vi "TX OOB Test Cases.vi"() -> (0 "error out":errorcluster, 2 "status":string, 3 "pass":bool)   [LabVIEW 2021]
uses:
  Common/Typedef/Plugin Status.ctl
  Common/Typedef/Plugin State.ctl
  Common/Typedef/Timing Statistics.ctl
  Common/Typedef/Timing Stats Base.ctl
  Common/Typedef/FIFO Statistics.ctl
  Common/Typedef/Simple Error.ctl
  Common/Typedef/Monitor Doubles.ctl
  Common/Typedef/Monitor U64.ctl
  Common/Typedef/Monitor I64.ctl
  CIFUtilities/CIFOutOfBand/CIFOutOfBand.lvclass/CIFOutOfBand.ctl
  OOB_Tx/Typedef/OOB Core Commands.ctl
  Common/Typedef/Plugin Overrides.ctl
  Common/Typedef/Timing Overrides.ctl
  CIFUtilities/CIFChannelMng/typedef/Channel List for OOB.ctl
  CIFUtilities/CIFChannels/Typedef/Direction.ctl
  OOB_Tx/Private/Command Settings.vi
  CIFUtilities/CIFOutOfBand/Accessors/Write Local OOB Data.vi
  CIFUtilities/CIFOutOfBand/Write OOB DVR.vi
  CIFUtilities/CIFOutOfBand/Utilities/Command to Bitwise Command.vi
  CIFUtilities/CIFOutOfBand/Accessors/Read Local OOB Data.vi
  CIFUtilities/CIFOutOfBand/Read OOB DVR.vi
  OOB_Tx/Private/Read Payload.vi
  OOB_Tx/CIFCoreOOB_Tx.lvclass
  D:/dev/CIF-LVCore/src/CIFUtilities/CIFOutOfBand/CIFOutOfBand.lvclass
  CIFUtilities/CIFOutOfBand/Init OOB.vi
  CIFUtilities/CIFOutOfBand/CIFOutOfBand.lvclass
  Common/CIFCoreCommon.lvlib
  CIFUtilities/CIFChannels/CIFChannels.lvclass
  CIFUtilities/CIFChannelMng/CIFChannelMng.lvclass
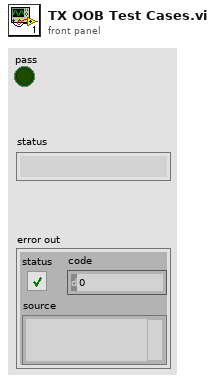
[diagram p1: front panel]
types:
  T1 = typedef "CIFCoreCommon.lvlib/Plugin Status.ctl" = cluster{"State":T2, "Timing Statistics (us)":T3, "FIFO Statistics (us)":T5, "error":T6, "Monitor Doubles":T7, "Monitor U64":T8, "Monitor I64":T9, "Cleanup":T4, "Create":i32, "Destroy":i32}
  T2 = typedef "CIFCoreCommon.lvlib/Plugin State.ctl" = enum32{"Null", "Creating", "Listening", "Running", "CleaningUp", "Destroying"}
  T3 = typedef "CIFCoreCommon.lvlib/Timing Statistics.ctl" = cluster{"Period":T4, "Wake Error":T4, "Execute":T4, "Housekeep":T4, "Idle":T4}
  T4 = typedef "CIFCoreCommon.lvlib/Timing Stats Base.ctl" = cluster{"Max":i32, "Min":i32}
  T5 = typedef "CIFCoreCommon.lvlib/FIFO Statistics.ctl" = cluster{"From T0":T4, "From Previous Plugin":T4, "Output Error":T4}
  T6 = typedef "CIFCoreCommon.lvlib/Simple Error.ctl" = cluster{"status":bool, "code":i32}
  T7 = typedef "CIFCoreCommon.lvlib/Monitor Doubles.ctl" = cluster{"1":dbl, "2":dbl, "3":dbl, "4":dbl}
  T8 = typedef "CIFCoreCommon.lvlib/Monitor U64.ctl" = cluster{"1":u64, "2":u64, "3":u64, "4":u64}
  T9 = typedef "CIFCoreCommon.lvlib/Monitor I64.ctl" = cluster{"1":i64, "2":i64, "3":i64, "4":i64}
  T10 = typedef "CIFCoreOOB_Tx.lvclass/OOB Core Commands.ctl" = enum8{"Status", "Overrides", "Channel List"}
  T11 = typedef "CIFChannelMng.lvclass/Channel List for OOB.ctl" = cluster{"Direction":T12, "Type":string, "Custom Config Data":variant, "Connected?":bool, "Connected Name":string}
  T12 = typedef "CIFChannels.lvclass/Direction.ctl" = enum16{"Publisher", "Subscriber"}
  T13 = typedef "CIFCoreCommon.lvlib/Plugin Overrides.ctl" = cluster{"Timing Overrides":T14}
  T14 = typedef "CIFCoreCommon.lvlib/Timing Overrides.ctl" = cluster{"Override Timing":bool, "Skip Sleep":bool, "Period (s)":dbl}
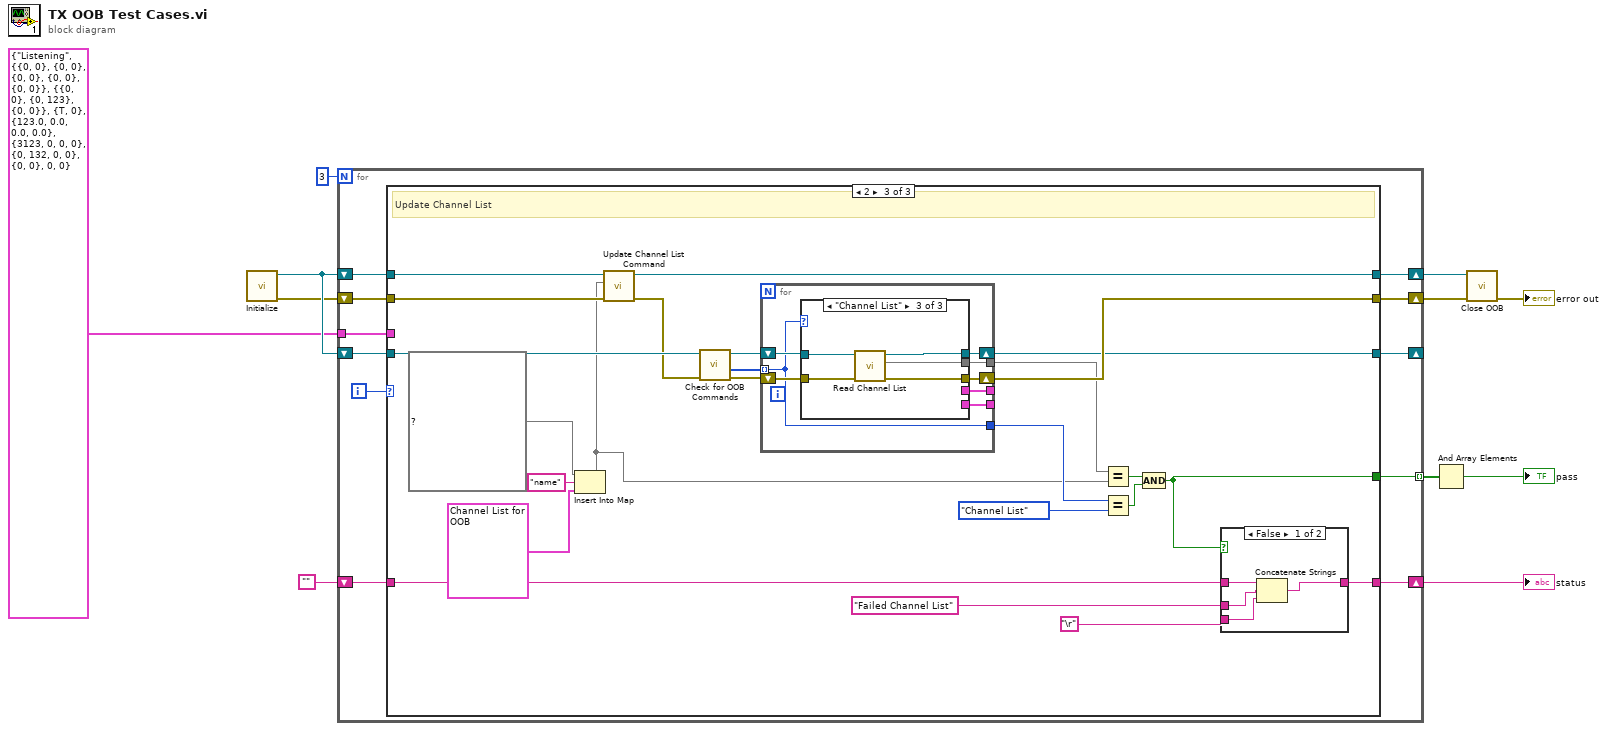
[diagram p0: block diagram]
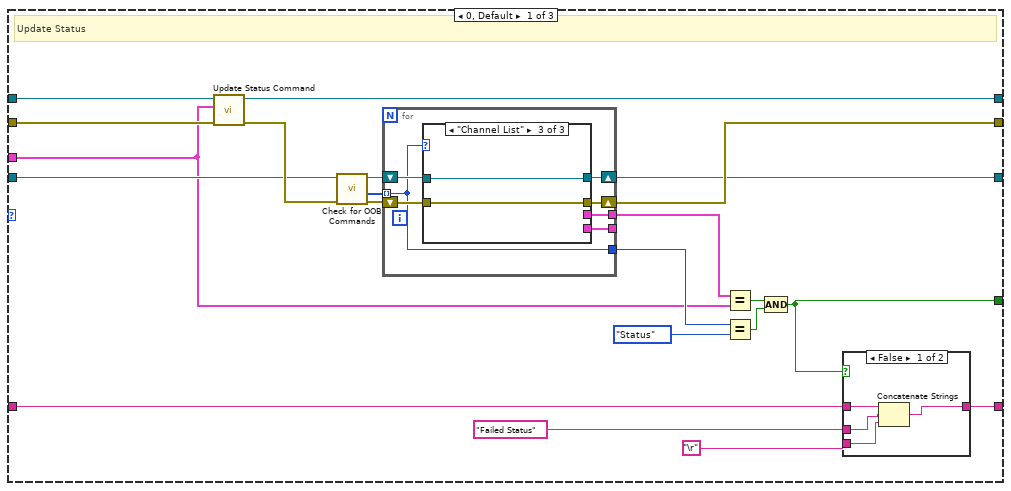
[diagram p2: hidden frame]
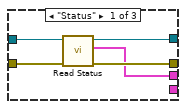
[diagram p3: hidden frame]
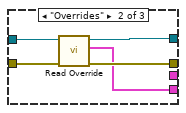
[diagram p4: hidden frame]
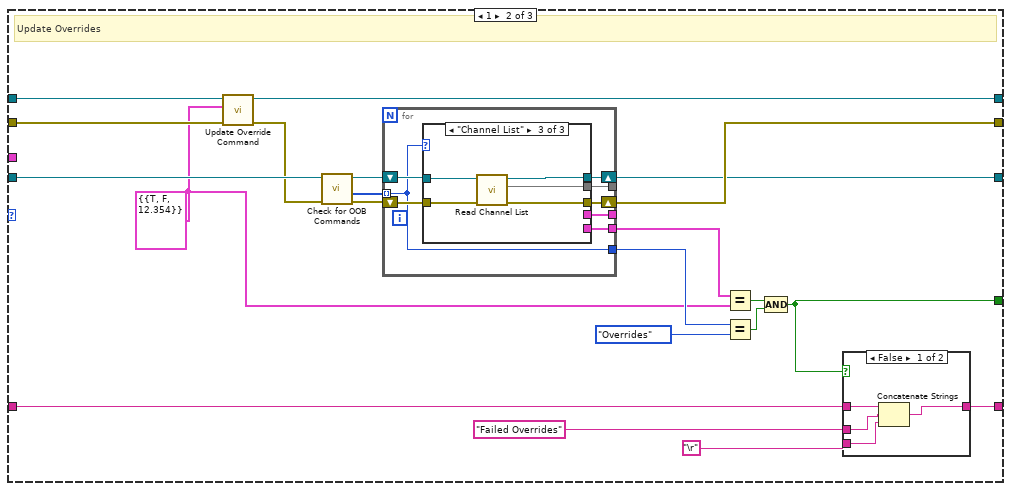
[diagram p6: hidden frame]
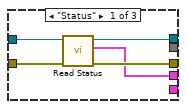
[diagram p7: hidden frame]
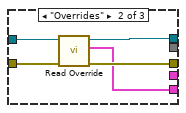
[diagram p8: hidden frame]
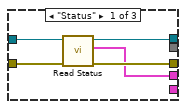
[diagram p10: hidden frame]
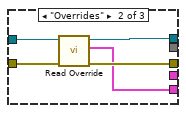
[diagram p11: hidden frame]
diagram:
  n1 = call "Initialize.vi"() -> ("error out"=w2:errorcluster, "CoreOOB_Tx out"=w3:refnum<class "CIFCoreOOB_Tx.lvclass">)  [unwired: 10 in]
  n2 = for {
    N: 3 -> [_]
    tunnel: [w22] -> w9 mode=indexing
    shift-right: [w19] -> w10
    shift-left: w2 -> [w21]
    shift-right: [w13] -> w11
    shift-left: w3 -> [w20]
    shift-right: [w12] -> _
    shift-left: w3 -> [w17]
    shift-right: [w15] -> w6
    shift-left: "" -> [w16]
    tunnel: T1 {"State"=enum."Listening", "Timing Statistics (us)"={"Period"={"Max"=0, "Min"=0}, "Wake Error"={"Max"=0, "Min"=0}, "Execute"={"Max"=0, "Min"=0}, "Housekeep"={"Max"=0, "Min"=0}, "Idle"={"Max"=0, "Min"=0}}, "FIFO Statistics (us)"={"From T0"={"Max"=0, "Min"=0}, "From Previous Plugin"={"Max"=0, "Min"=123}, "Output Error"={"Max"=0, "Min"=0}}, "error"={"status"=TRUE, "code"=0}, "Monitor Doubles"={"1"=123.0, "2"=0.0, "3"=0.0, "4"=0.0}, "Monitor U64"={"1"=3123, "2"=0, "3"=0, "4"=0}, "Monitor I64"={"1"=0, "2"=132, "3"=0, "4"=0}, "Cleanup"={"Max"=0, "Min"=0}, "Create"=0, "Destroy"=0} ("Status") -> [w14]
    i -> [w18]
    n3 = case shown="2" w18 {
      tunnel: [w35 w80 w132] -> w22
      tunnel: w21 -> [w30 w71 w124]
      tunnel: w20 -> [w32 w72 w125]
      tunnel: [w43 w88 w140] -> w19
      tunnel: [w31 w69 w123] -> w13
      tunnel: w17 -> [w28 w78 w130]
      tunnel: [w42 w87 w139] -> w12
      tunnel: w16 -> [w41 w86 w138]
      tunnel: [w40 w85 w137] -> w15
      tunnel: w14 -> [w24 _ _]
      frame 0, Default {
        # "Update Status"
        n4 = call "Update Status Command.vi"("error in"=w30, "Status"=w24, "CoreOOB_Tx in"=w32) -> ("error out"=w29:errorcluster, "CoreOOB_Tx out"=w31:refnum<class "CIFCoreOOB_Tx.lvclass">)  [unwired: 7 in]
        n5 = call "Check for OOB Commands.vi"("error in (no error)"=w29, "CoreOOB_Tx in"=w28) -> ("error out"=w27:errorcluster, "Commands"=w25:T10[], "CoreOOB_Tx out"=w26:refnum<class "CIFCoreOOB_Tx.lvclass">)  [unwired: 6 in, 1 out]
        n6 = for {
          tunnel: w25 -> [w45] mode=indexing
          shift-right: [w50] -> w43
          shift-left: w27 -> [w48]
          shift-right: [w49] -> w42
          shift-left: w26 -> [w47]
          tunnel: [w46] -> w34
          tunnel: [w45] -> w33
          tunnel: [w44] -> _
          n7 = case shown="\"Channel List\"" w45 {
            tunnel: w47 -> [w55 w59 w62]
            tunnel: w48 -> [w54 w60 w61]
            tunnel: [w53 w58 w62] -> w49
            tunnel: [w52 w57 w61] -> w50
            tunnel: [w51 _ _] -> w46
            tunnel: [_ w56 _] -> w44
            frame "Status" {
              n8 = call "Read Status.vi"("error in"=w54, "CoreOOB_Tx in"=w55) -> ("error out"=w52:errorcluster, "Status"=w51:T1, "CoreOOB_Tx out"=w53:refnum<class "CIFCoreOOB_Tx.lvclass">)  [unwired: 7 in]
            }
            frame "Overrides" {
              n9 = call "Read Override.vi"("error in"=w60, "CoreOOB_Tx in"=w59) -> ("error out"=w57:errorcluster, "Plugin Overrides"=w56:T13, "CoreOOB_Tx out"=w58:refnum<class "CIFCoreOOB_Tx.lvclass">)  [unwired: 7 in]
            }
            frame "Channel List" {
            }
          }
        }
        n10 = Equal?(x=w34, y=w24) -> (x = y?=w37:bool)
        n11 = Equal?(x=w33, y=OOB_Core_Commands."Status") -> (x = y?=w36:bool)
        n12 = Compound Arithmetic op=AND(w37, w36) -> (w35:bool)
        n13 = case shown="False" w35 {
          tunnel: w41 -> [w66 w67]
          tunnel: [w63 w67] -> w40
          tunnel: "Failed Status" -> [w65 _]
          tunnel: "\r" -> [w64 _]
          frame False {
            n14 = Concatenate Strings(w66, w65, w64) -> (w63:string)
          }
          frame True {
          }
        }
      }
      frame 1 {
        w68 = T13 {"Timing Overrides"={"Override Timing"=TRUE, "Skip Sleep"=FALSE, "Period (s)"=12.354}} ("Plugin Overrides")
        # "Update Overrides"
        n15 = call "Update Override Command.vi"("error in"=w71, "Plugin Overrides"=w68, "CoreOOB_Tx in"=w72) -> ("error out"=w70:errorcluster, "CoreOOB_Tx out"=w69:refnum<class "CIFCoreOOB_Tx.lvclass">)  [unwired: 7 in]
        n16 = call "Check for OOB Commands.vi"("error in (no error)"=w70, "CoreOOB_Tx in"=w78) -> ("error out"=w77:errorcluster, "Commands"=w75:T10[], "CoreOOB_Tx out"=w76:refnum<class "CIFCoreOOB_Tx.lvclass">)  [unwired: 6 in, 1 out]
        n17 = for {
          tunnel: w75 -> [w91] mode=indexing
          shift-right: [w96] -> w88
          shift-left: w77 -> [w94]
          shift-right: [w95] -> w87
          shift-left: w76 -> [w93]
          tunnel: [w92] -> _
          tunnel: [w91] -> w79
          tunnel: [w90] -> w73
          tunnel: [w89] -> _
          n18 = case shown="\"Channel List\"" w91 {
            tunnel: w93 -> [w101 w105 w111]
            tunnel: w94 -> [w100 w106 w110]
            tunnel: [w99 w104 w109] -> w95
            tunnel: [w98 w103 w108] -> w96
            tunnel: [w97 _ _] -> w92
            tunnel: [_ w102 _] -> w90
            tunnel: [_ _ w107] -> w89
            frame "Status" {
              n19 = call "Read Status.vi"("error in"=w100, "CoreOOB_Tx in"=w101) -> ("error out"=w98:errorcluster, "Status"=w97:T1, "CoreOOB_Tx out"=w99:refnum<class "CIFCoreOOB_Tx.lvclass">)  [unwired: 7 in]
            }
            frame "Overrides" {
              n20 = call "Read Override.vi"("error in"=w106, "CoreOOB_Tx in"=w105) -> ("error out"=w103:errorcluster, "Plugin Overrides"=w102:T13, "CoreOOB_Tx out"=w104:refnum<class "CIFCoreOOB_Tx.lvclass">)  [unwired: 7 in]
            }
            frame "Channel List" {
              n21 = call "Read Channel List.vi"("error in"=w110, "CoreOOB_Tx in"=w111) -> ("error out"=w108:errorcluster, "Channel List"=w107:map{string, T11}, "CoreOOB_Tx out"=w109:refnum<class "CIFCoreOOB_Tx.lvclass">)  [unwired: 7 in]
            }
          }
        }
        n22 = Equal?(x=w73, y=w68) -> (x = y?=w82:bool)
        n23 = Equal?(x=w79, y=OOB_Core_Commands."Overrides") -> (x = y?=w81:bool)
        n24 = Compound Arithmetic op=AND(w82, w81) -> (w80:bool)
        n25 = case shown="False" w80 {
          tunnel: w86 -> [w115 w116]
          tunnel: [w112 w116] -> w85
          tunnel: "Failed Overrides" -> [w114 _]
          tunnel: "\r" -> [w113 _]
          frame False {
            n26 = Concatenate Strings(w115, w114, w113) -> (w112:string)
          }
          frame True {
          }
        }
      }
      frame 2 {
        # "Update Channel List"
        n27 = Insert Into Map(map in=map{string, T11} {} ("Channel List"), key="name", value=T11 {"Direction"=enum."Publisher", "Type"="data", "Custom Config Data"=variant(string "name"), "Connected?"=FALSE, "Connected Name"=""}) -> (map out=w118:map{string, T11})  [unwired: 2 out]
        n28 = call "Update Channel List Command.vi"("error in"=w124, "Channel List"=w118, "CoreOOB_Tx in"=w125) -> ("error out"=w122:errorcluster, "CoreOOB_Tx out"=w123:refnum<class "CIFCoreOOB_Tx.lvclass">)  [unwired: 7 in]
        n29 = call "Check for OOB Commands.vi"("error in (no error)"=w122, "CoreOOB_Tx in"=w130) -> ("error out"=w129:errorcluster, "Commands"=w127:T10[], "CoreOOB_Tx out"=w128:refnum<class "CIFCoreOOB_Tx.lvclass">)  [unwired: 6 in, 1 out]
        n30 = for {
          tunnel: w127 -> [w143] mode=indexing
          shift-right: [w148] -> w140
          shift-left: w129 -> [w146]
          shift-right: [w147] -> w139
          shift-left: w128 -> [w145]
          tunnel: [w144] -> _
          tunnel: [w143] -> w131
          tunnel: [w142] -> _
          tunnel: [w141] -> w117
          n31 = case shown="\"Channel List\"" w143 {
            tunnel: w145 -> [w153 w157 w163]
            tunnel: w146 -> [w152 w158 w162]
            tunnel: [w151 w156 w161] -> w147
            tunnel: [w150 w155 w160] -> w148
            tunnel: [w149 _ _] -> w144
            tunnel: [_ w154 _] -> w142
            tunnel: [_ _ w159] -> w141
            frame "Status" {
              n32 = call "Read Status.vi"("error in"=w152, "CoreOOB_Tx in"=w153) -> ("error out"=w150:errorcluster, "Status"=w149:T1, "CoreOOB_Tx out"=w151:refnum<class "CIFCoreOOB_Tx.lvclass">)  [unwired: 7 in]
            }
            frame "Overrides" {
              n33 = call "Read Override.vi"("error in"=w158, "CoreOOB_Tx in"=w157) -> ("error out"=w155:errorcluster, "Plugin Overrides"=w154:T13, "CoreOOB_Tx out"=w156:refnum<class "CIFCoreOOB_Tx.lvclass">)  [unwired: 7 in]
            }
            frame "Channel List" {
              n34 = call "Read Channel List.vi"("error in"=w162, "CoreOOB_Tx in"=w163) -> ("error out"=w160:errorcluster, "Channel List"=w159:map{string, T11}, "CoreOOB_Tx out"=w161:refnum<class "CIFCoreOOB_Tx.lvclass">)  [unwired: 7 in]
            }
          }
        }
        n35 = Equal?(x=w117, y=w118) -> (x = y?=w134:bool)
        n36 = Equal?(x=w131, y=OOB_Core_Commands."Channel List") -> (x = y?=w133:bool)
        n37 = Compound Arithmetic op=AND(w134, w133) -> (w132:bool)
        n38 = case shown="False" w132 {
          tunnel: w138 -> [w167 w168]
          tunnel: [w164 w168] -> w137
          tunnel: "Failed Channel List" -> [w166 _]
          tunnel: "\r" -> [w165 _]
          frame False {
            n39 = Concatenate Strings(w167, w166, w165) -> (w164:string)
          }
          frame True {
          }
        }
      }
    }
  }
  "status" <- w6
  n40 = And Array Elements(Boolean array=w9) -> (logical AND=→"pass":bool)
  n41 = call "Close OOB.vi"("error in"=w10, "OOB in"=w11) -> ("error out"=→"error out":errorcluster)  [unwired: 9 in]
